vi "laser_control.vi"(0 "VISA resource name":refnum<visa-resource-name>, 1 "write or read":u16(ring) items=["read", "write"], 2 "laser number":u16(ring)=3 items=["laser No 0", "laser No 1", "laser No 2", "laser No 3", "laser No 4", "laser No 5"], 5 "laser mode":u16(ring) items=["OFF", "ON", "RISING", "FALLING", "CAMERA"], 7 "duration":u32(slide) max=65535 step=1 scale=0.0..65535.0 scale format="%u us", 9 "sequence":bool[](array[boolean])=[FALSE, FALSE, FALSE, FALSE, FALSE, FALSE, FALSE, FALSE, FALSE, FALSE, FALSE, FALSE, FALSE, FALSE, FALSE, FALSE]) -> (4 "VISA out":refnum<visa-resource-name>, 6 "laser mode 2":u16(ring) items=["OFF", "ON", "RISING", "FALLING", "CAMERA"], 8 "duration 2":u32(slide) max=65535 step=1 scale=0.0..65535.0 scale format="%u us", 10 "Boolean array":bool[](array[boolean]))   [LabVIEW 2021]
panel:
  out "sequence read string":string
  out "sequence read string answer":string
  out "sequence write string":string
  out "duration read string":string
  out "duration read string answer":string
  out "duration write string":string
  out "mode read string answer":string
  out "mode read string":string
  out "mode write string":string
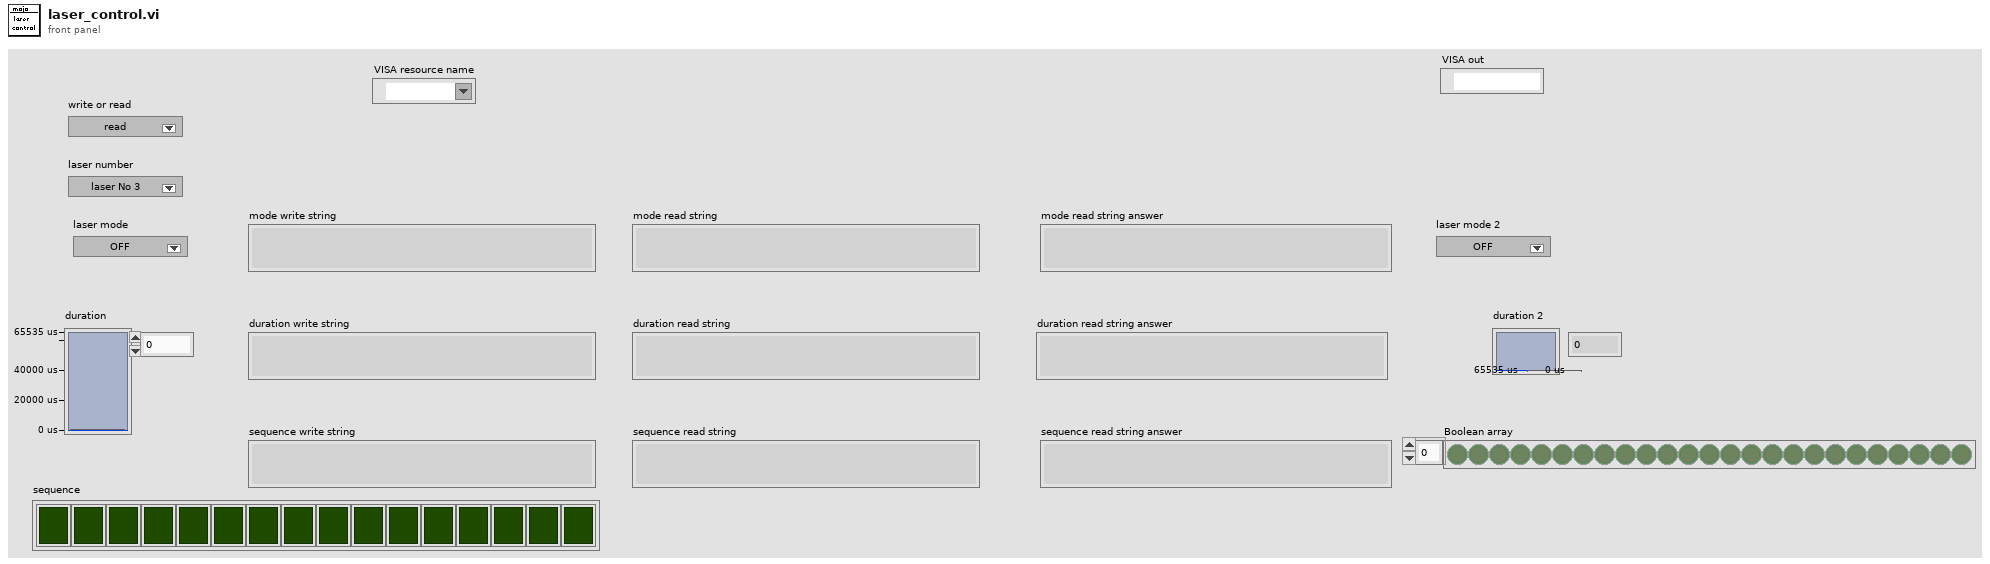
[diagram p1: front panel]
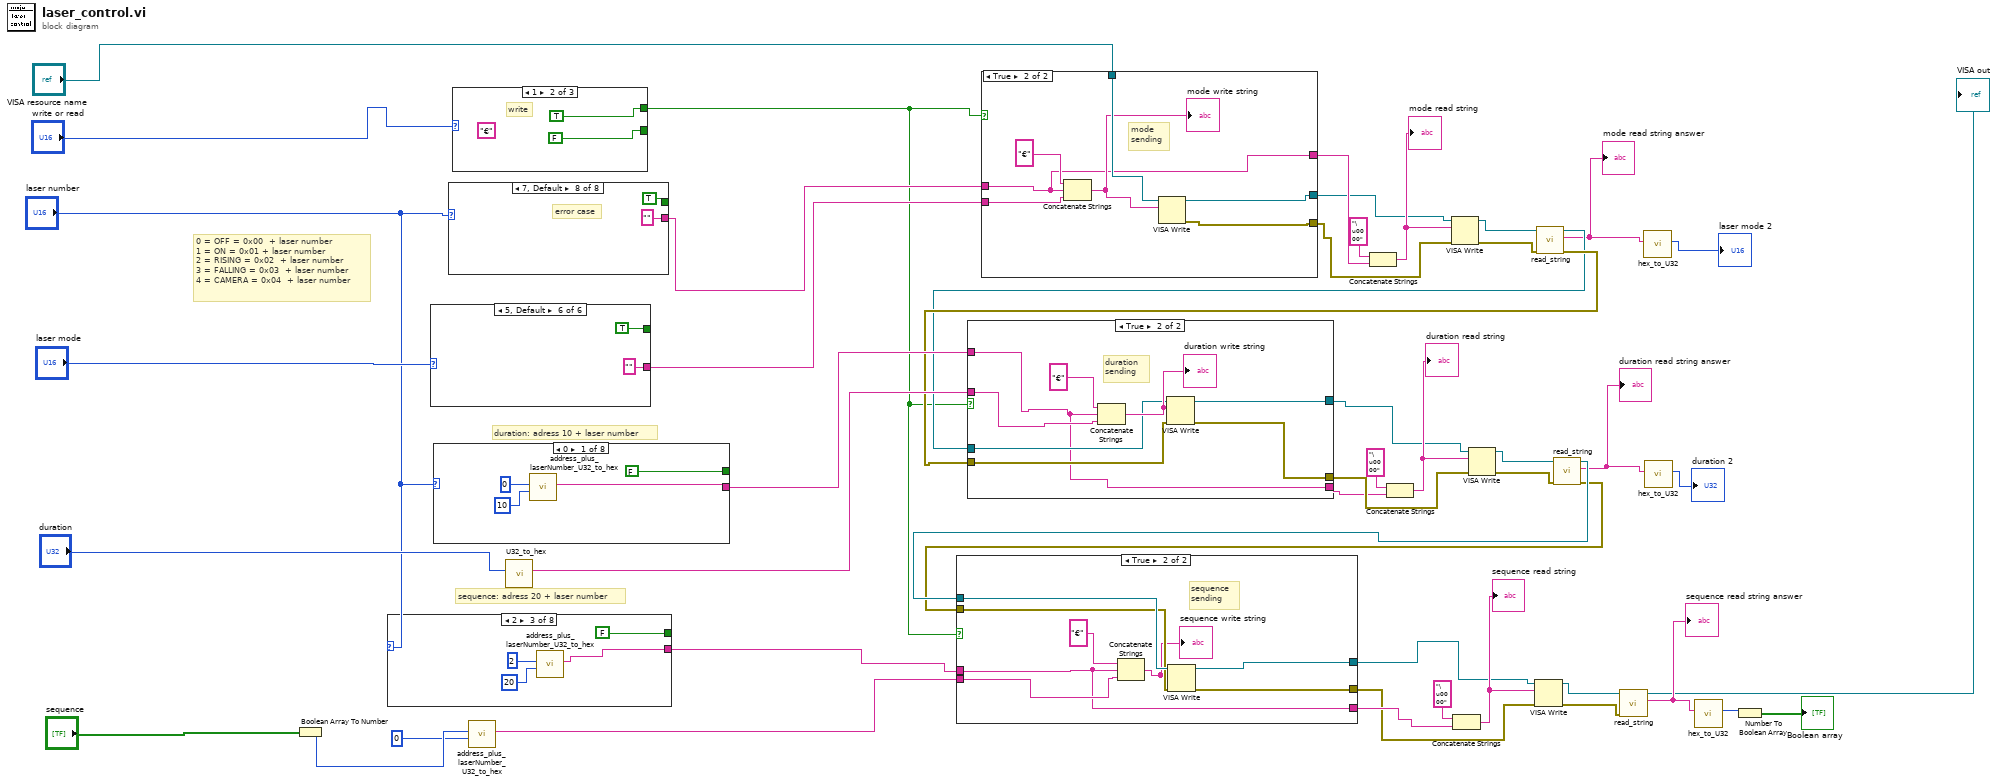
[diagram p0: block diagram]
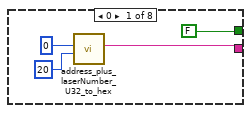
[diagram p4: hidden frame]
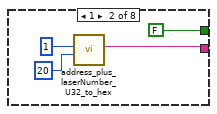
[diagram p5: hidden frame]
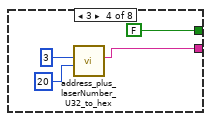
[diagram p6: hidden frame]
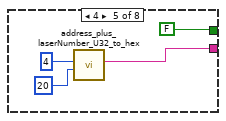
[diagram p7: hidden frame]
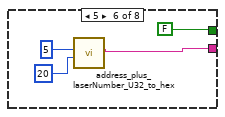
[diagram p8: hidden frame]
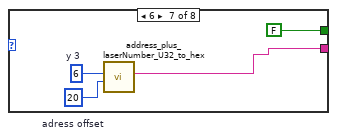
[diagram p9: hidden frame]
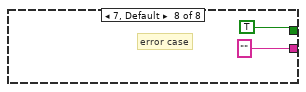
[diagram p10: hidden frame]
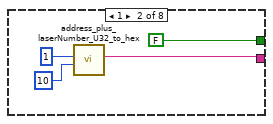
[diagram p11: hidden frame]
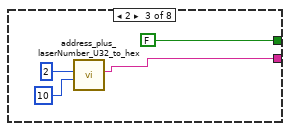
[diagram p12: hidden frame]
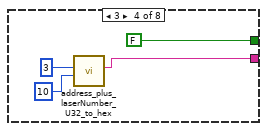
[diagram p13: hidden frame]
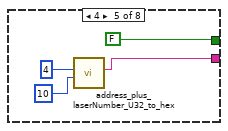
[diagram p14: hidden frame]
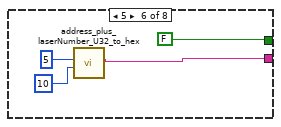
[diagram p15: hidden frame]
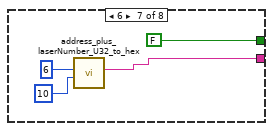
[diagram p16: hidden frame]
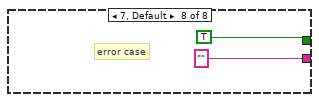
[diagram p17: hidden frame]
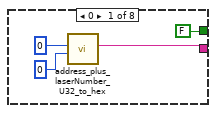
[diagram p19: hidden frame]
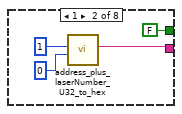
[diagram p20: hidden frame]
diagram:
  # "sequence: adress 20 + laser number"
  # "duration: adress 10 + laser number"
  # "0 = OFF = 0x00  + laser number\n1 = ON = 0x01 + laser number\n2 = RISING = 0x02  + laser number\n3 = FALLING = 0x03  + laser number\n4 = CAMERA = 0x04  + laser number"
  n1 = Boolean Array To Number(Boolean array="sequence") -> (number=w45:u32)
  n2 = case shown="2" "laser number" {
    tunnel: [w49 w53 w57 w61 w65 w69 w73 "" ("string 5")] -> w22
    tunnel: [FALSE FALSE FALSE FALSE FALSE FALSE FALSE TRUE] -> _
    frame 0 {
      n3 = call "address_plus_laserNumber_U32_to_hex.vi"("adress offset"=u32 20, "y 3"=u32 0) -> ("string 5"=w49:string)  [unwired: 8 in]
    }
    frame 1 {
      n4 = call "address_plus_laserNumber_U32_to_hex.vi"("adress offset"=u32 20, "y 3"=u32 1) -> ("string 5"=w53:string)  [unwired: 8 in]
    }
    frame 2 {
      n5 = call "address_plus_laserNumber_U32_to_hex.vi"("adress offset"=u32 20, "y 3"=u32 2) -> ("string 5"=w57:string)  [unwired: 8 in]
    }
    frame 3 {
      n6 = call "address_plus_laserNumber_U32_to_hex.vi"("adress offset"=u32 20, "y 3"=u32 3) -> ("string 5"=w61:string)  [unwired: 8 in]
    }
    frame 4 {
      n7 = call "address_plus_laserNumber_U32_to_hex.vi"("adress offset"=u32 20, "y 3"=u32 4) -> ("string 5"=w65:string)  [unwired: 8 in]
    }
    frame 5 {
      n8 = call "address_plus_laserNumber_U32_to_hex.vi"("adress offset"=u32 20, "y 3"=u32 5) -> ("string 5"=w69:string)  [unwired: 8 in]
    }
    frame 6 {
      w74 = u32 6  # y 3
      w75 = u32 20  # adress offset
      n9 = call "address_plus_laserNumber_U32_to_hex.vi"("adress offset"=w75, "y 3"=w74) -> ("string 5"=w73:string)  [unwired: 8 in]
    }
    frame 7, Default {
      # "error case"
    }
  }
  n10 = case shown="5, Default" "laser mode" {
    tunnel: [w79 w84 w88 w92 w96 "" ("string 5")] -> w38
    tunnel: [FALSE FALSE FALSE FALSE FALSE TRUE] -> _
    frame 0 {
      n11 = call "address_plus_laserNumber_U32_to_hex.vi"("adress offset"=u32 0, "y 3"=u32 0) -> ("string 5"=w79:string)  [unwired: 8 in]
    }
    frame 1 {
      n12 = call "address_plus_laserNumber_U32_to_hex.vi"("adress offset"=u32 0, "y 3"=u32 1) -> ("string 5"=w84:string)  [unwired: 8 in]
    }
    frame 2 {
      n13 = call "address_plus_laserNumber_U32_to_hex.vi"("adress offset"=u32 0, "y 3"=u32 2) -> ("string 5"=w88:string)  [unwired: 8 in]
    }
    frame 3 {
      n14 = call "address_plus_laserNumber_U32_to_hex.vi"("adress offset"=u32 0, "y 3"=u32 3) -> ("string 5"=w92:string)  [unwired: 8 in]
    }
    frame 4 {
      n15 = call "address_plus_laserNumber_U32_to_hex.vi"("adress offset"=u32 0, "y 3"=u32 4) -> ("string 5"=w96:string)  [unwired: 8 in]
    }
    frame 5, Default {
    }
  }
  n16 = case shown="0" "laser number" {
    tunnel: [w101 w105 w109 w113 w117 w121 w125 "" ("string 5")] -> w32
    tunnel: [FALSE FALSE FALSE FALSE FALSE FALSE FALSE TRUE] -> _
    frame 0 {
      n17 = call "address_plus_laserNumber_U32_to_hex.vi"("adress offset"=u32 10, "y 3"=u32 0) -> ("string 5"=w101:string)  [unwired: 8 in]
    }
    frame 1 {
      n18 = call "address_plus_laserNumber_U32_to_hex.vi"("adress offset"=u32 10, "y 3"=u32 1) -> ("string 5"=w105:string)  [unwired: 8 in]
    }
    frame 2 {
      n19 = call "address_plus_laserNumber_U32_to_hex.vi"("adress offset"=u32 10, "y 3"=u32 2) -> ("string 5"=w109:string)  [unwired: 8 in]
    }
    frame 3 {
      n20 = call "address_plus_laserNumber_U32_to_hex.vi"("adress offset"=u32 10, "y 3"=u32 3) -> ("string 5"=w113:string)  [unwired: 8 in]
    }
    frame 4 {
      n21 = call "address_plus_laserNumber_U32_to_hex.vi"("adress offset"=u32 10, "y 3"=u32 4) -> ("string 5"=w117:string)  [unwired: 8 in]
    }
    frame 5 {
      n22 = call "address_plus_laserNumber_U32_to_hex.vi"("adress offset"=u32 10, "y 3"=u32 5) -> ("string 5"=w121:string)  [unwired: 8 in]
    }
    frame 6 {
      n23 = call "address_plus_laserNumber_U32_to_hex.vi"("adress offset"=u32 10, "y 3"=u32 6) -> ("string 5"=w125:string)  [unwired: 8 in]
    }
    frame 7, Default {
      # "error case"
    }
  }
  n24 = case shown="7, Default" "laser number" {
    tunnel: [w131 w135 w139 w143 w147 w151 w155 "" ("string 5")] -> w39
    tunnel: [FALSE FALSE FALSE FALSE FALSE FALSE FALSE TRUE] -> _
    frame 0 {
      n25 = call "address_plus_laserNumber_U32_to_hex.vi"("adress offset"=u32 0, "y 3"=u32 0) -> ("string 5"=w131:string)  [unwired: 8 in]
    }
    frame 1 {
      n26 = call "address_plus_laserNumber_U32_to_hex.vi"("adress offset"=u32 0, "y 3"=u32 1) -> ("string 5"=w135:string)  [unwired: 8 in]
    }
    frame 2 {
      n27 = call "address_plus_laserNumber_U32_to_hex.vi"("adress offset"=u32 0, "y 3"=u32 2) -> ("string 5"=w139:string)  [unwired: 8 in]
    }
    frame 3 {
      n28 = call "address_plus_laserNumber_U32_to_hex.vi"("adress offset"=u32 0, "y 3"=u32 3) -> ("string 5"=w143:string)  [unwired: 8 in]
    }
    frame 4 {
      n29 = call "address_plus_laserNumber_U32_to_hex.vi"("adress offset"=u32 0, "y 3"=u32 4) -> ("string 5"=w147:string)  [unwired: 8 in]
    }
    frame 5 {
      n30 = call "address_plus_laserNumber_U32_to_hex.vi"("adress offset"=u32 0, "y 3"=u32 5) -> ("string 5"=w151:string)  [unwired: 8 in]
    }
    frame 6 {
      n31 = call "address_plus_laserNumber_U32_to_hex.vi"("adress offset"=u32 0, "y 3"=u32 6) -> ("string 5"=w155:string)  [unwired: 8 in]
    }
    frame 7, Default {
      # "error case"
    }
  }
  n32 = case shown="1" "write or read" {
    tunnel: [w161 TRUE FALSE] -> w12
    tunnel: [w161 FALSE TRUE] -> _
    frame 0 {
      w161 = FALSE
    }
    frame 1 {
      (unwired) "€" ("hex")
      # "write"
    }
    frame 2, Default {
      # "error"
    }
  }
  n33 = call "address_plus_laserNumber_U32_to_hex.vi"("adress offset"=u32 0, "y 3"=w45) -> ("string 5"=w21:string)  [unwired: 8 in]
  n34 = call "U32_to_hex.vi"("y 3"="duration") -> ("string 5"=w31:string)  [unwired: 9 in]
  n35 = case shown="True" w12 {
    tunnel: w39 -> [w167 w171]
    tunnel: "VISA resource name" -> [w166 w173]
    tunnel: [w167 w171] -> w40
    tunnel: w38 -> [_ w170]
    tunnel: [w166 w169] -> w34
    tunnel: [_ w168] -> w33
    frame False {
    }
    frame True {
      # "mode \nsending"
      n36 = Concatenate Strings("€" ("string"), w171, w170) -> (w172:string)
      "mode write string" <- w172
      n37 = VISA Write(VISA resource name=w173, write buffer=w172) -> (VISA resource name out=w169:refnum<visa-resource-name>, error out=w168:errorcluster)  [unwired: 1 in, 1 out]
    }
  }
  n38 = Concatenate Strings("\u0000" ("string"), w40) -> (w37:string)
  "mode read string" <- w37
  n39 = VISA Write(VISA resource name=w34, write buffer=w37, error in (no error)=w33) -> (VISA resource name out=w36:refnum<visa-resource-name>, error out=w35:errorcluster)  [unwired: 1 out]
  n40 = call "read_string.vi"("error in (no error)"=w35, "VISA resource name 2"=w36) -> ("error out"=w30:errorcluster, "read buffer"=w3:string, "VISA resource name"=w24:refnum<visa-resource-name>)  [unwired: 7 in]
  "mode read string answer" <- w3
  n41 = case shown="True" w12 {
    tunnel: w32 -> [w175 w178]
    tunnel: w31 -> [_ w184]
    tunnel: w30 -> [w176 w183]
    tunnel: [w176 w181] -> w25
    tunnel: w24 -> [w177 w180]
    tunnel: [w177 w179] -> w23
    tunnel: [w175 w178] -> w18
    frame False {
    }
    frame True {
      # "duration \nsending"
      n42 = Concatenate Strings("€" ("string"), w178, w184) -> (w182:string)
      "duration write string" <- w182
      n43 = VISA Write(VISA resource name=w180, write buffer=w182, error in (no error)=w183) -> (VISA resource name out=w179:refnum<visa-resource-name>, error out=w181:errorcluster)  [unwired: 1 out]
    }
  }
  n44 = Concatenate Strings("\u0000" ("string"), w18) -> (w27:string)
  "duration read string" <- w27
  n45 = VISA Write(VISA resource name=w23, write buffer=w27, error in (no error)=w25) -> (VISA resource name out=w28:refnum<visa-resource-name>, error out=w29:errorcluster)  [unwired: 1 out]
  n46 = call "read_string.vi"("error in (no error)"=w29, "VISA resource name 2"=w28) -> ("error out"=w19:errorcluster, "read buffer"=w8:string, "VISA resource name"=w20:refnum<visa-resource-name>)  [unwired: 7 in]
  "duration read string answer" <- w8
  n47 = case shown="True" w12 {
    tunnel: w22 -> [w186 w190]
    tunnel: w21 -> [_ w195]
    tunnel: w20 -> [w188 w194]
    tunnel: w19 -> [w187 w193]
    tunnel: [w188 w191] -> w13
    tunnel: [w186 w190] -> w11
    tunnel: [w187 w189] -> w10
    frame False {
    }
    frame True {
      # "sequence \nsending"
      n48 = Concatenate Strings("€" ("string"), w190, w195) -> (w192:string)
      "sequence write string" <- w192
      n49 = VISA Write(VISA resource name=w194, write buffer=w192, error in (no error)=w193) -> (VISA resource name out=w191:refnum<visa-resource-name>, error out=w189:errorcluster)  [unwired: 1 out]
    }
  }
  n50 = Concatenate Strings("\u0000" ("string"), w11) -> (w16:string)
  "sequence read string" <- w16
  n51 = VISA Write(VISA resource name=w13, write buffer=w16, error in (no error)=w10) -> (VISA resource name out=w15:refnum<visa-resource-name>, error out=w14:errorcluster)  [unwired: 1 out]
  n52 = call "read_string.vi"("error in (no error)"=w14, "VISA resource name 2"=w15) -> ("read buffer"=w7:string, "VISA resource name"=→"VISA out":refnum<visa-resource-name>)  [unwired: 7 in, 1 out]
  "sequence read string answer" <- w7
  n53 = call "hex_to_U32.vi"("hex"=w3) -> ("U32"=→"laser mode 2":u32)  [unwired: 9 in]
  n54 = call "hex_to_U32.vi"("hex"=w8) -> ("U32"=→"duration 2":u32)  [unwired: 9 in]
  n55 = call "hex_to_U32.vi"("hex"=w7) -> ("U32"=w6:u32)  [unwired: 9 in]
  n56 = Number To Boolean Array(number=w6) -> (Boolean array=→"Boolean array":bool[])
